vi "Two dimensional Array Demo.vi"() -> ()   [LabVIEW 2016]
panel:
  out "数组":dbl[][](array[numeric])
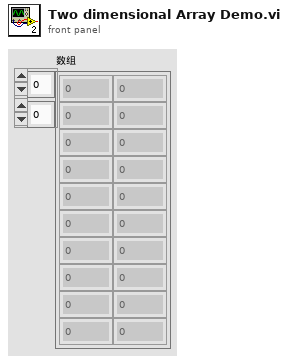
[diagram p1: front panel]
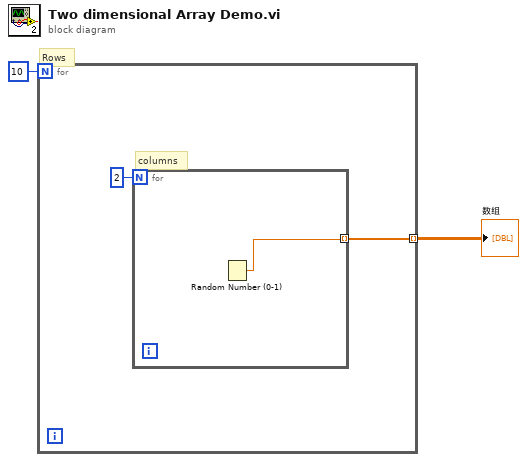
[diagram p0: block diagram]
diagram:
  # "Rows"
  n1 = for {
    N: 10 -> [_]
    tunnel: [w3] -> w1 mode=indexing
    # "columns"
    n2 = for {
      N: 2 -> [_]
      tunnel: [w5] -> w3 mode=indexing
      n3 = Random Number (0-1)() -> (number: 0 to 1=w5:dbl)
    }
  }
  "数组" <- w1
